vi "SWERVE_DRIVE_BEGIN.vi"(8 "error in":errorcluster) -> (0 "error out":errorcluster)   [LabVIEW 2023]
uses:
  <vilib>/Rock Robotics/WPI/ThirdParty/Phoenix-LabVIEW/Motor Controller/Controls/CTRE_Phoenix_MotorControl_TalonFXInvertType.ctl
  <vilib>/Rock Robotics/WPI/ThirdParty/Phoenix-LabVIEW/Pigeon IMU/CTRE_PigeonIMU_TareType.ctl
  <vilib>/Rock Robotics/WPI/ThirdParty/JAS_Junk/TrajLib/Trajectory_Library.lvlib
  SWERVE_DRIVE_GLOBALS.vi
  <vilib>/Rock Robotics/WPI/ThirdParty/JAS_Junk/TrajLib/Enum/DCMOTOR_TYPES_ENUM.ctl
  <vilib>/Rock Robotics/WPI/ThirdParty/Phoenix-LabVIEW/CANCoder/Controls/CTRE_Phoenix_CANcoder_StatusFrame.ctl
  <vilib>/Rock Robotics/WPI/ThirdParty/Phoenix-LabVIEW/CANCoder/Controls/CTRE_Phoenix_CANcoder_SensorInitializationStrategy.ctl
  <vilib>/Rock Robotics/WPI/ThirdParty/Phoenix-LabVIEW/Motor Controller/Controls/CTRE_Phoenix_MotorControl_FeedbackDevice_TalonFX.ctl
  <vilib>/Rock Robotics/WPI/ThirdParty/Phoenix-LabVIEW/Motor Controller/Controls/CTRE_Phoenix_MotorControl_NeutralMode.ctl
  <vilib>/Rock Robotics/WPI/ThirdParty/REV Robotics/REVLib/Typedef/Spark MAX Idle Mode.ctl
  <vilib>/Rock Robotics/WPI/ThirdParty/Phoenix-LabVIEW/Motor Controller/Controls/CTRE_Phoenix_MotorControl_StatorCurrentLimitConfiguration.ctl
  <vilib>/Analysis/Matrix/Datatypes/RealMatrix.ctl
  <vilib>/Analysis/Matrix/NI_Matrix.lvlib
  <vilib>/Rock Robotics/WPI/ThirdParty/Phoenix6/setters/TalonFX_SetSensorPosition.vi
  <vilib>/Rock Robotics/Network Tables/NT Write Variant.vi
  <vilib>/Rock Robotics/WPI/ThirdParty/JAS_Junk/TrajLib/TypeDef/DCMOTOR_SIM_SIMULATION_PARAMS.ctl
  <vilib>/Rock Robotics/WPI/ThirdParty/REV Robotics/REVLib/SubVI/Public/SPARK Open Brushless.vi
  <vilib>/Rock Robotics/WPI/ThirdParty/REV Robotics/REVLib/Typedef/Closed Loop Voltage Mode.ctl
  <vilib>/Rock Robotics/WPI/ThirdParty/REV Robotics/REVLib/Typedef/SPARK PID Gains.ctl
  <vilib>/Rock Robotics/WPI/ThirdParty/REV Robotics/REVLib/Typedef/SPARK Feedback Sensor.ctl
  <vilib>/Rock Robotics/WPI/ThirdParty/REV Robotics/REVLib/SubVI/Public/SPARK Configure Closed Loop MAXMotion.vi
  <vilib>/Rock Robotics/WPI/ThirdParty/REV Robotics/REVLib/SubVI/Public/SPARK Configure Closed Loop Voltage Mode.vi
  <vilib>/Rock Robotics/WPI/ThirdParty/REV Robotics/REVLib/SubVI/Public/SPARK Configure Closed Loop Gains.vi
  <vilib>/Rock Robotics/WPI/ThirdParty/REV Robotics/REVLib/SubVI/Public/SPARK Configure Basic Idle Mode.vi
  <vilib>/Rock Robotics/WPI/ThirdParty/REV Robotics/REVLib/SubVI/Public/SPARK Configure Closed Loop Basic.vi
  <vilib>/Rock Robotics/WPI/ThirdParty/REV Robotics/REVLib/SubVI/Public/SPARK Configure Power Smart Current Limit.vi
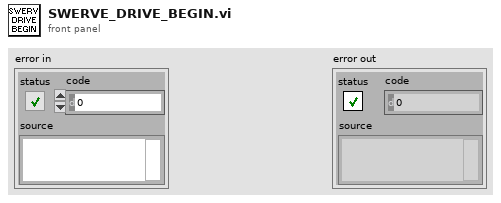
[diagram p1: front panel]
types:
  T1 = enum16{"Talon FX, P5", "Talon FX, P6", "SPARK MAX"}
  T2 = typedef "NI_Matrix.lvlib/RealMatrix.ctl" = dbl[][]
  T3 = typedef "CTRE_Phoenix_MotorControl_TalonFXInvertType.ctl" = enum16{"Counter-Clockwise", "Clockwise"}
  T4 = typedef "Trajectory_Library.lvlib/DCMOTOR_TYPES_ENUM.ctl" = enum16{"CIM", "AndyMark 9015", "Andy Mark RS 775 125", "Bag", "BaneBots RS 550", "BaneBots RS 775", "Falcon 500", "Mini CIM", "NEO", "NEO 550", "Romi BuiltIn", "Vex 775 Pro", "Snow Blower AM 2235A", "Bosch Seat AM 3493", "Falcon 500 FOC", "Kraken X60", "Kraken X60 FOC", "NEO Vortex"}
  T5 = typedef "Trajectory_Library.lvlib/DCMOTOR.CTL" = cluster{"nominalVoltage_Volts":dbl, "StallTorque_NM":dbl, "StallCurrent_Amps":dbl, "FreeCurrent_Amps":dbl, "FreeSpeed_RadPerSec":dbl, "R_Ohms":dbl, "KvINV_RadPerSecPerVolt":dbl, "Kt_NMPerAmp":dbl, "L_H":dbl, "Jr_KgM2":dbl}
  T6 = cluster{"Future Proof Configs":bool, "MotorOutputInverted":u16, "MotorOutputNeutralMode":u16, "MotorOutputDutyCycleNeutralDeadband":dbl, "MotorOutputPeakForwardDutyCycle":dbl, "MotorOutputPeakReverseDutyCycle":dbl, "MotorOutputControlTimesyncFreqHz":dbl, "CurrentLimitsStatorCurrentLimit":dbl, "CurrentLimitsStatorCurrentLimitEnable":bool, "CurrentLimitsSupplyCurrentLimit":dbl, "CurrentLimitsSupplyCurrentLimitEnable":bool, "CurrentLimitsSupplyCurrentLowerLimit":dbl, "CurrentLimitsSupplyCurrentLowerTime":dbl, "VoltageSupplyVoltageTimeConstant":dbl, "VoltagePeakForwardVoltage":dbl, "VoltagePeakReverseVoltage":dbl, "TorqueCurrentPeakForwardTorqueCurrent":dbl, "TorqueCurrentPeakReverseTorqueCurrent":dbl, "TorqueCurrentTorqueNeutralDeadband":dbl, "FeedbackFeedbackRotorOffset":dbl, "FeedbackSensorToMechanismRatio":dbl, "FeedbackRotorToSensorRatio":dbl, "FeedbackFeedbackSensorSource":u16, "FeedbackFeedbackRemoteSensorID":i16, "FeedbackVelocityFilterTimeConstant":dbl, "DifferentialSensorsDifferentialSensorSource":u16, "DifferentialSensorsDifferentialTalonFXSensorID":i16, "DifferentialSensorsDifferentialRemoteSensorID":i16, "DifferentialConstantsPeakDifferentialDutyCycle":dbl, "DifferentialConstantsPeakDifferentialVoltage":dbl, "DifferentialConstantsPeakDifferentialTorqueCurrent":dbl, "OpenLoopRampsDutyCycleOpenLoopRampPeriod":dbl, "OpenLoopRampsVoltageOpenLoopRampPeriod":dbl, "OpenLoopRampsTorqueOpenLoopRampPeriod":dbl, "ClosedLoopRampsDutyCycleClosedLoopRampPeriod":dbl, "ClosedLoopRampsVoltageClosedLoopRampPeriod":dbl, "ClosedLoopRampsTorqueClosedLoopRampPeriod":dbl, "HardwareLimitSwitchForwardLimitType":u16, "HardwareLimitSwitchForwardLimitAutosetPositionEnable":bool, "HardwareLimitSwitchForwardLimitAutosetPositionValue":dbl, "HardwareLimitSwitchForwardLimitEnable":bool, "HardwareLimitSwitchForwardLimitSource":u16, "HardwareLimitSwitchForwardLimitRemoteSensorID":i16, "HardwareLimitSwitchReverseLimitType":u16, "HardwareLimitSwitchReverseLimitAutosetPositionEnable":bool, "HardwareLimitSwitchReverseLimitAutosetPositionValue":dbl, "HardwareLimitSwitchReverseLimitEnable":bool, "HardwareLimitSwitchReverseLimitSource":u16, "HardwareLimitSwitchReverseLimitRemoteSensorID":i16, "AudioBeepOnBoot":bool, "AudioBeepOnConfig":bool, "AudioAllowMusicDurDisable":bool, "SoftwareLimitSwitchForwardSoftLimitEnable":bool, "SoftwareLimitSwitchReverseSoftLimitEnable":bool, "SoftwareLimitSwitchForwardSoftLimitThreshold":dbl, "SoftwareLimitSwitchReverseSoftLimitThreshold":dbl, "MotionMagicMotionMagicCruiseVelocity":dbl, "MotionMagicMotionMagicAcceleration":dbl, "MotionMagicMotionMagicJerk":dbl, "MotionMagicMotionMagicExpo_kV":dbl, "MotionMagicMotionMagicExpo_kA":dbl, "CustomParamsCustomParam0":i16, "CustomParamsCustomParam1":i16, "ClosedLoopGeneralContinuousWrap":bool, "Slot0kP":dbl, "Slot0kI":dbl, "Slot0kD":dbl, "Slot0kS":dbl, "Slot0kV":dbl, "Slot0kA":dbl, "Slot0kG":dbl, "Slot0GravityType":u16, "Slot0StaticFeedforwardSign":u16, "Slot1kP":dbl, "Slot1kI":dbl, "Slot1kD":dbl, "Slot1kS":dbl, "Slot1kV":dbl, "Slot1kA":dbl, "Slot1kG":dbl, "Slot1GravityType":u16, "Slot1StaticFeedforwardSign":u16, "Slot2kP":dbl, "Slot2kI":dbl, "Slot2kD":dbl, "Slot2kS":dbl, "Slot2kV":dbl, "Slot2kA":dbl, "Slot2kG":dbl, "Slot2GravityType":u16, "Slot2StaticFeedforwardSign":u16}
  T7 = typedef "Trajectory_Library.lvlib/DCMOTOR_SIM_SIMULATION_PARAMS.ctl" = cluster{"Pos Sim Std Dev Rotations":dbl, "Vel Sim Std Dev RPM":dbl}
  T8 = typedef "CTRE_Phoenix_MotorControl_StatorCurrentLimitConfiguration.ctl" = cluster{"Enable?":bool, "Current Limit":dbl, "Threshold Current":dbl, "Threshold Time":dbl}
  T9 = typedef "CTRE_Phoenix_MotorControl_NeutralMode.ctl" = enum8{"EEPROMSetting", "Override to Coast", "Override to Brake"}
  T10 = typedef "SPARK Feedback Sensor.ctl" = enum16{"No Sensor", "Primary Encoder", "Analog Sensor", "Alternate or External Encoder", "Duty Cycle Sensor"}
  T11 = typedef "Spark MAX Idle Mode.ctl" = enum16{"Coast", "Brake"}
  T12 = typedef "SPARK PID Gains.ctl" = cluster{"kP":dbl, "kI":dbl, "kD":dbl}
  T13 = typedef "Closed Loop Voltage Mode.ctl" = enum16{"Disabled", "Voltage Output", "Voltage Compensation"}
  T14 = typedef "CTRE_Phoenix_CANcoder_SensorInitializationStrategy.ctl" = enum16{"Boot To Zero", "Boot To Absolute Position"}
  T15 = typedef "Trajectory_Library.lvlib/LINEAR_SYSTEM.ctl" = cluster{"m_A":T2, "m_B":T2, "m_C":T2, "m_D":T2, "States":i32, "Inputs":i32, "Outputs":i32}
  T16 = typedef "Trajectory_Library.lvlib/DCMOTOR_SIM.ctl" = cluster{"LinearSystemSim":T17, "GearBox":T5, "Gearing":dbl}
  T17 = typedef "Trajectory_Library.lvlib/LINEAR_SYSTEM_SIM.ctl" = cluster{"m_Plant":T15, "m_X":T2, "m_Y":T2, "m_U":T2, "MeasureStdDev":T2}
  T18 = typedef "CTRE_PigeonIMU_TareType.ctl" = u8
  T19 = typedef "CTRE_Phoenix_MotorControl_FeedbackDevice_TalonFX.ctl" = i8
  T20 = typedef "WPI_MotorControlDeviceRef.ctl" = cluster{"DeviceStatus":errorcluster, "Type":T21, "PWM":cluster{"PWM Channel":T22, "DeadBand":T23}, "CAN":cluster{"Device Number":u8, "SetOutput VI Ref":variant, "GetOutput VI Ref":variant, "Enable VI Ref":variant, "Disable VI Ref":variant, "Data":variant}, "Invert":bool, "DIO PWM":cluster{"PWM \"Enable\" Channel":T22, "DIOChannel":T24, "PWM Rate":dbl}}
  T21 = typedef "WPI_MotorControlType.ctl" = enum16{"PWM", "CAN", "DIO PWM"}
  T22 = typedef "FPGA_DIOPWMChannel.ctl" = enum8{"PWM 0", "PWM 1", "PWM 2", "PWM 3", "PWM 4", "PWM 5", "PWM 6", "PWM 7", "PWM 8", "PWM 9", "PWM MXP 0", "PWM MXP 1", "PWM MXP 2", "PWM MXP 3", "PWM MXP 4", "PWM MXP 5", "PWM MXP 6", "PWM MXP 7", "PWM MXP 8", "PWM MXP 9", "Invalid"}
  T23 = typedef "WPI_PWMDeadband.ctl" = cluster{"Name":string, "maxPositivePwm":i32, "minPositivePwm":i32, "centerPwm":i32, "maxNegativePwm":i32, "minNegativePwm":i32, "angularRange":u16}
  T24 = typedef "FPGA_DIOChannel.ctl" = enum8{"DIO 0", "DIO 1", "DIO 2", "DIO 3", "DIO 4", "DIO 5", "DIO 6", "DIO 7", "DIO 8", "DIO 9", "DIO MXP 0", "DIO MXP 1", "DIO MXP 2", "DIO MXP 3", "DIO MXP 4", "DIO MXP 5", "DIO MXP 6", "DIO MXP 7", "DIO MXP 8", "DIO MXP 9", "DIO MXP 10", "DIO MXP 11", "DIO MXP 12", "DIO MXP 13", "DIO MXP 14", "DIO MXP 15", "SPI Port CS1", "SPI Port CS2", "SPI Port CS3", "SPI Port MISO", "SPI Port MOSI", "Invalid"}
  T25 = typedef "DeviceReference.ctl" = cluster{"CANbus Name":string, "Device Encoding":u32, "Device Name":string}
  T26 = typedef "CTRE_Phoenix_CANcoder_StatusFrame.ctl" = u32
  T27 = typedef "CTRE_Phoenix_CANcoder_DeviceRef.ctl" = cluster{"DeviceStatus":errorcluster, "Device Number":u8, "Handle":u64, "UsageFrame":u32, "Library Path":path}
  T28 = typedef "CTRE_PigeonIMU_DeviceRef.ctl" = cluster{"DeviceStatus":errorcluster, "Device Number":u8, "Type":T29, "Device ID":u32, "Handle":u64, "UsageFrame":u32, "Library Path":path}
  T29 = typedef "CTRE_PigeonIMU_ConnectionType.ctl" = u32
  T30 = typedef "Trajectory_Library.lvlib/TRANSLATION2D.ctl" = cluster{"X":dbl, "Y":dbl}
  T31 = typedef "Trajectory_Library.lvlib/SWERVE_DRIVE_KINEMATICS.ctl" = cluster{"NumModules":i32, "InverseKinematics":T2, "ForwardKinematics":T2, "Modules":T30[], "PrevCoR":T30, "SavedModuleStates":T32[]}
  T32 = typedef "Trajectory_Library.lvlib/SWERVE_DRIVE_MODULE_STATE.ctl" = cluster{"Speed":dbl, "Angle":T33}
  T33 = typedef "Trajectory_Library.lvlib/ROTATION2D.ctl" = cluster{"VALUE":dbl, "COS":dbl, "SIN":dbl}
  T34 = typedef "Trajectory_Library.lvlib/SWERVE_DRIVE_MODULE_POSITION.ctl" = cluster{"Distance":dbl, "Angle":T33, "P":bool}
  T35 = typedef "Trajectory_Library.lvlib/POSE2D.ctl" = cluster{"TRANSLATION":T30, "ROTATION":T33}
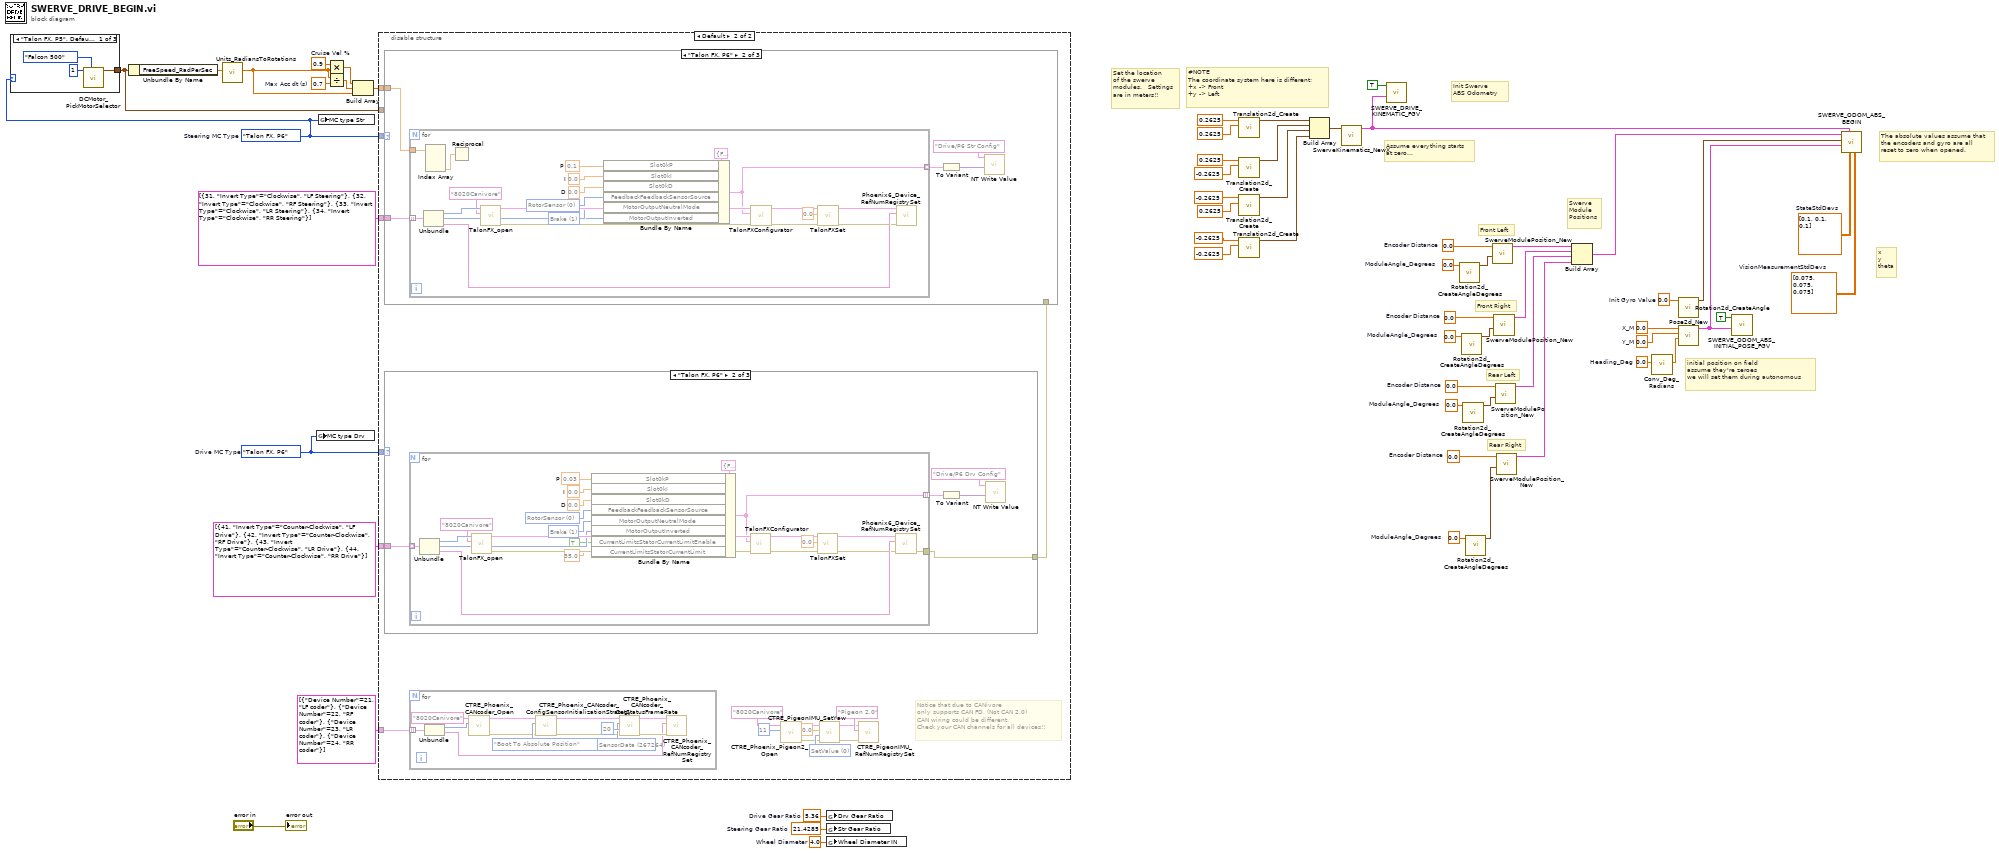
[diagram p0: block diagram]
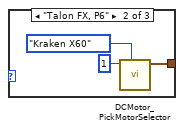
[diagram p2: hidden frame]
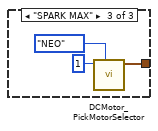
[diagram p3: hidden frame]
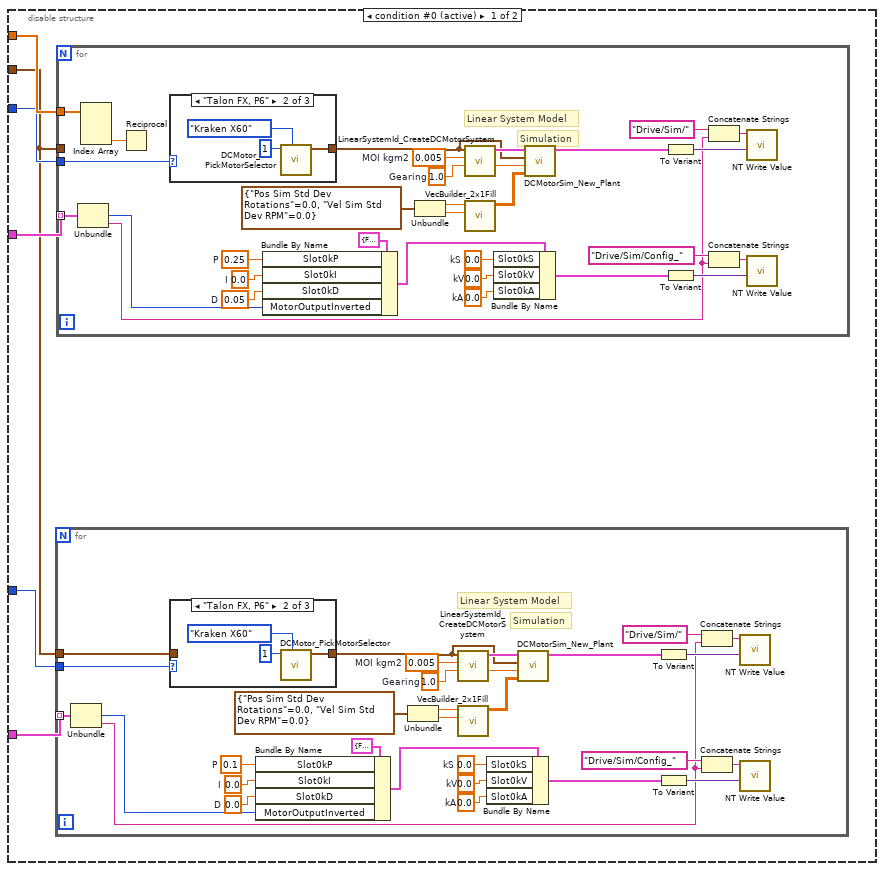
[diagram p4: hidden frame]
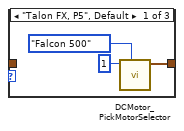
[diagram p5: hidden frame]
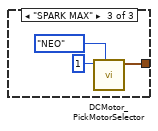
[diagram p6: hidden frame]
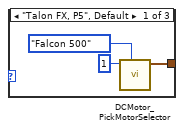
[diagram p7: hidden frame]
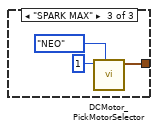
[diagram p8: hidden frame]
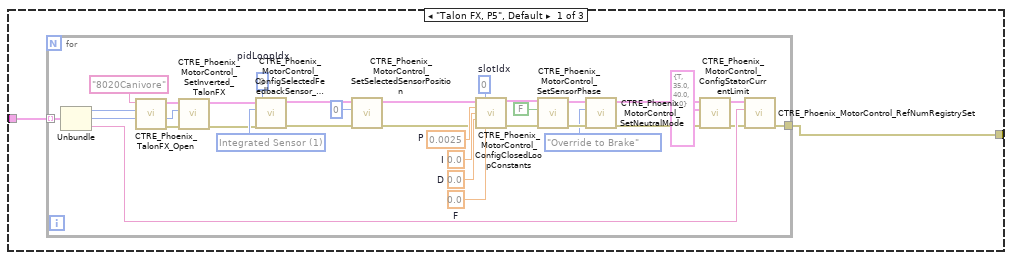
[diagram p9: hidden frame]
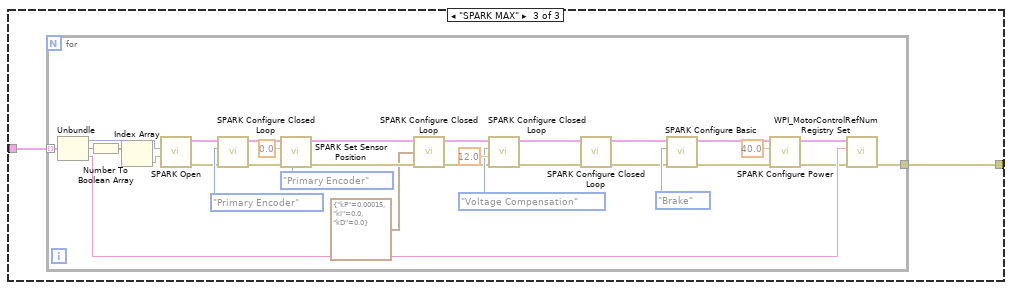
[diagram p10: hidden frame]
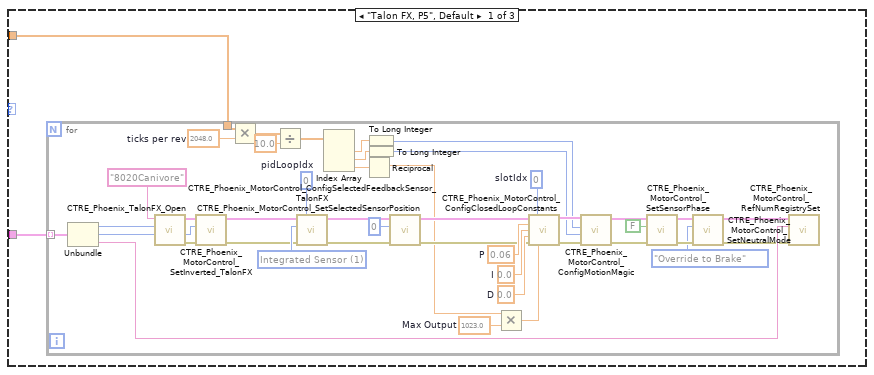
[diagram p11: hidden frame]
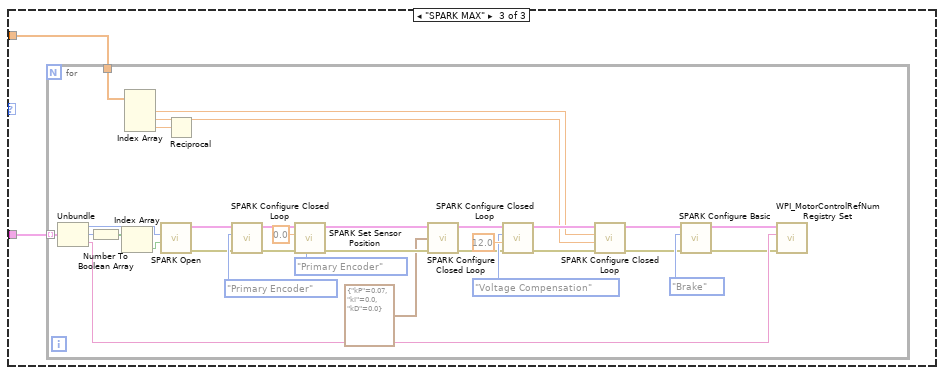
[diagram p12: hidden frame]
diagram:
  w3 = 4.0  # Wheel Diameter
  w5 = T1."Talon FX, P6"  # Drive MC Type
  w1 = T1."Talon FX, P6"  # Steering MC Type
  w9 = 0.7  # Max Acc dt (s)
  w8 = 0.9  # Cruise Vel %
  w55 = T2 [[0.075], [0.075], [0.075]]  # VisionMeasurementStdDevs
  w54 = T2 [[0.1], [0.1], [0.1]]  # StateStdDevs
  w50 = 0.0  # Init Gyro Value
  w51 = 0.0  # Heading_Deg
  w49 = 0.0  # Y_M
  w48 = 0.0  # X_M
  w35 = 0.0  # ModuleAngle_Degrees
  w37 = 0.0  # Encoder Distance
  w38 = 0.0  # ModuleAngle_Degrees
  w40 = 0.0  # Encoder Distance
  w41 = 0.0  # ModuleAngle_Degrees
  w43 = 0.0  # Encoder Distance
  w45 = 0.0  # ModuleAngle_Degrees
  w47 = 0.0  # Encoder Distance
  w4 = 21.4285  # Steering Gear Ratio
  w28 = 5.36  # Drive Gear Ratio
  # "x\ny\ntheta"
  # "Init Swerve\nABS Odometry"
  # "initial position on field\nassume they're zeroes\nwe will set them during autonomous"
  # "The absolute values assume that\nthe encoders and gyro are all\nreset to zero when opened."
  # "Assume everything starts\nat zero..."
  # "Front Left"
  # "Swerve\nModule\nPositions"
  # "Rear Right"
  # "Rear Left"
  # "Front Right"
  # "#NOTE\nThe coordinate system here is different;\n+x -> Front\n+y -> Left"
  # "Set the location\nof the swerve \nmodules.   Settings\nare in meters!!"
  n1 = case shown="\"Talon FX, P5\", Default" w1 {
    tunnel: [w61 w64 w67] -> w2
    frame "Talon FX, P5", Default {
      n2 = call <vilib>:"DCMotor_PickMotorSelector.vi"("DCMOTOR_TYPES"=DCMOTOR_TYPES_ENUM."Falcon 500", "Num Motors"=1) -> ("DCMOTOR"=w61:T5)  [unwired: 9 in]
    }
    frame "Talon FX, P6" {
      n3 = call <vilib>:"DCMotor_PickMotorSelector.vi"("DCMOTOR_TYPES"=DCMOTOR_TYPES_ENUM."Kraken X60", "Num Motors"=1) -> ("DCMOTOR"=w64:T5)  [unwired: 9 in]
    }
    frame "SPARK MAX" {
      n4 = call <vilib>:"DCMotor_PickMotorSelector.vi"("DCMOTOR_TYPES"=DCMOTOR_TYPES_ENUM."NEO", "Num Motors"=1) -> ("DCMOTOR"=w67:T5)  [unwired: 9 in]
    }
  }
  n5 = Unbundle By Name(w2) -> ("FreeSpeed_RadPerSec"=w29:dbl)
  n6 = call <vilib>:"Units_RadiansToRotations.vi"("Radians"=w29) -> ("Rotations"=w7:dbl)  [unwired: 10 in]
  n7 = global write "SWERVE_DRIVE_GLOBALS.vi" "MC type Drv"(w5) -> ()
  n8 = global write "SWERVE_DRIVE_GLOBALS.vi" "MC type Str"(w1) -> ()
  n9 = Multiply(x=w8, y=w7) -> (x*y=w10:dbl)
  n10 = Divide(x=w7, y=w9) -> (x/y=w11:dbl)
  n11 = Build Array(w10, w11, w7) -> (w6:dbl[])
  n12 = disable-structure shown="Default" {
    disable-tunnel: cluster{i32, "Invert Type":T3, string}[] [{31, "Invert Type"=enum."Clockwise", "LF Steering"}, {32, "Invert Type"=enum."Clockwise", "RF Steering"}, {33, "Invert Type"=enum."Clockwise", "LR Steering"}, {34, "Invert Type"=enum."Clockwise", "RR Steering"}] ("Array") -> [w74 w166]
    disable-tunnel: cluster{"Device Number":u8, string}[] [{"Device Number"=21, "LF coder"}, {"Device Number"=22, "RF coder"}, {"Device Number"=23, "LR coder"}, {"Device Number"=24, "RR coder"}] ("CANcoder ref") -> [_ w165]
    disable-tunnel: cluster{i32, "Invert Type":T3, string}[] [{41, "Invert Type"=enum."Counter-Clockwise", "LF Drive"}, {42, "Invert Type"=enum."Counter-Clockwise", "RF Drive"}, {43, "Invert Type"=enum."Counter-Clockwise", "LR Drive"}, {44, "Invert Type"=enum."Counter-Clockwise", "RR Drive"}] ("Array") -> [w73 w155]
    disable-tunnel: w6 -> [w72 w154]
    disable-tunnel: w5 -> [w70 w153]
    disable-tunnel: w1 -> [w71 w152]
    disable-tunnel: w2 -> [w69 _]
    frame condition #0 (active) {
      n13 = for {
        tunnel: w73 -> [w78] mode=indexing
        tunnel: w70 -> [w77]
        tunnel: w69 -> [w76]
        w84 = 0.0  # kA
        w85 = 0.0  # kV
        w86 = 0.0  # kS
        w89 = 0.0  # D
        w90 = 0.0  # I
        w91 = 0.1  # P
        w95 = 1.0  # Gearing
        w94 = 0.005  # MOI kgm2
        # "Simulation"
        # "Linear System Model"
        n14 = Unbundle(w78) -> ("Invert Type"=w88:T3, w79:string)  [unwired: 1 out]
        n15 = case shown="\"Talon FX, P6\"" w77 {
          tunnel: w76 -> [_ _ _]
          tunnel: [w105 w108 w111] -> w93
          frame "Talon FX, P5", Default {
            n16 = call <vilib>:"DCMotor_PickMotorSelector.vi"("DCMOTOR_TYPES"=DCMOTOR_TYPES_ENUM."Falcon 500", "Num Motors"=1) -> ("DCMOTOR"=w105:T5)  [unwired: 9 in]
          }
          frame "Talon FX, P6" {
            n17 = call <vilib>:"DCMotor_PickMotorSelector.vi"("DCMOTOR_TYPES"=DCMOTOR_TYPES_ENUM."Kraken X60", "Num Motors"=1) -> ("DCMOTOR"=w108:T5)  [unwired: 9 in]
          }
          frame "SPARK MAX" {
            n18 = call <vilib>:"DCMotor_PickMotorSelector.vi"("DCMOTOR_TYPES"=DCMOTOR_TYPES_ENUM."NEO", "Num Motors"=1) -> ("DCMOTOR"=w111:T5)  [unwired: 9 in]
          }
        }
        n19 = Bundle By Name(cluster=T6 {"Future Proof Configs"=FALSE, "MotorOutputInverted"=0, "MotorOutputNeutralMode"=0, "MotorOutputDutyCycleNeutralDeadband"=0.0, "MotorOutputPeakForwardDutyCycle"=1.0, "MotorOutputPeakReverseDutyCycle"=-1.0, "MotorOutputControlTimesyncFreqHz"=0.0, "CurrentLimitsStatorCurrentLimit"=120.0, "CurrentLimitsStatorCurrentLimitEnable"=TRUE, "CurrentLimitsSupplyCurrentLimit"=70.0, "CurrentLimitsSupplyCurrentLimitEnable"=TRUE, "CurrentLimitsSupplyCurrentLowerLimit"=40.0, "CurrentLimitsSupplyCurrentLowerTime"=1.0, "VoltageSupplyVoltageTimeConstant"=0.0, "VoltagePeakForwardVoltage"=16.0, "VoltagePeakReverseVoltage"=-16.0, "TorqueCurrentPeakForwardTorqueCurrent"=800.0, "TorqueCurrentPeakReverseTorqueCurrent"=-800.0, "TorqueCurrentTorqueNeutralDeadband"=0.0, "FeedbackFeedbackRotorOffset"=0.0, "FeedbackSensorToMechanismRatio"=1.0, "FeedbackRotorToSensorRatio"=1.0, "FeedbackFeedbackSensorSource"=0, "FeedbackFeedbackRemoteSensorID"=0, "FeedbackVelocityFilterTimeConstant"=0.0, "DifferentialSensorsDifferentialSensorSource"=0, "DifferentialSensorsDifferentialTalonFXSensorID"=0, "DifferentialSensorsDifferentialRemoteSensorID"=0, "DifferentialConstantsPeakDifferentialDutyCycle"=2.0, "DifferentialConstantsPeakDifferentialVoltage"=32.0, "DifferentialConstantsPeakDifferentialTorqueCurrent"=1600.0, "OpenLoopRampsDutyCycleOpenLoopRampPeriod"=0.0, "OpenLoopRampsVoltageOpenLoopRampPeriod"=0.0, "OpenLoopRampsTorqueOpenLoopRampPeriod"=0.0, "ClosedLoopRampsDutyCycleClosedLoopRampPeriod"=0.0, "ClosedLoopRampsVoltageClosedLoopRampPeriod"=0.0, "ClosedLoopRampsTorqueClosedLoopRampPeriod"=0.0, "HardwareLimitSwitchForwardLimitType"=0, "HardwareLimitSwitchForwardLimitAutosetPositionEnable"=FALSE, "HardwareLimitSwitchForwardLimitAutosetPositionValue"=0.0, "HardwareLimitSwitchForwardLimitEnable"=TRUE, "HardwareLimitSwitchForwardLimitSource"=0, "HardwareLimitSwitchForwardLimitRemoteSensorID"=0, "HardwareLimitSwitchReverseLimitType"=0, "HardwareLimitSwitchReverseLimitAutosetPositionEnable"=FALSE, "HardwareLimitSwitchReverseLimitAutosetPositionValue"=0.0, "HardwareLimitSwitchReverseLimitEnable"=TRUE, "HardwareLimitSwitchReverseLimitSource"=0, "HardwareLimitSwitchReverseLimitRemoteSensorID"=0, "AudioBeepOnBoot"=TRUE, "AudioBeepOnConfig"=TRUE, "AudioAllowMusicDurDisable"=FALSE, "SoftwareLimitSwitchForwardSoftLimitEnable"=FALSE, "SoftwareLimitSwitchReverseSoftLimitEnable"=FALSE, "SoftwareLimitSwitchForwardSoftLimitThreshold"=0.0, "SoftwareLimitSwitchReverseSoftLimitThreshold"=0.0, "MotionMagicMotionMagicCruiseVelocity"=0.0, "MotionMagicMotionMagicAcceleration"=0.0, "MotionMagicMotionMagicJerk"=0.0, "MotionMagicMotionMagicExpo_kV"=0.12, "MotionMagicMotionMagicExpo_kA"=0.1, "CustomParamsCustomParam0"=0, "CustomParamsCustomParam1"=0, "ClosedLoopGeneralContinuousWrap"=FALSE, "Slot0kP"=0.0, "Slot0kI"=0.0, "Slot0kD"=0.0, "Slot0kS"=0.0, "Slot0kV"=0.0, "Slot0kA"=0.0, "Slot0kG"=0.0, "Slot0GravityType"=0, "Slot0StaticFeedforwardSign"=0, "Slot1kP"=0.0, "Slot1kI"=0.0, "Slot1kD"=0.0, "Slot1kS"=0.0, "Slot1kV"=0.0, "Slot1kA"=0.0, "Slot1kG"=0.0, "Slot1GravityType"=0, "Slot1StaticFeedforwardSign"=0, "Slot2kP"=0.0, "Slot2kI"=0.0, "Slot2kD"=0.0, "Slot2kS"=0.0, "Slot2kV"=0.0, "Slot2kA"=0.0, "Slot2kG"=0.0, "Slot2GravityType"=0, "Slot2StaticFeedforwardSign"=0} ("DeviceConfiguration"), "Slot0kP"=w91, "Slot0kI"=w90, "Slot0kD"=w89, "MotorOutputInverted"=w88) -> (w87:T6)
        n20 = Unbundle(T7 {"Pos Sim Std Dev Rotations"=0.0, "Vel Sim Std Dev RPM"=0.0} ("DCMOTORSim_Simulation_Params")) -> ("Pos Sim Std Dev Rotations"=w100:dbl, "Vel Sim Std Dev RPM"=w99:dbl)
        n21 = call <vilib>:"LinearSystemId_CreateDCMotorSystem.vi"("G"=w95, "jKgMetersSquared"=w94, "DCMOTOR"=w93) -> ("Linearsystem"=w103:T15)  [unwired: 7 in, 1 out]
        n22 = call <vilib>:"VecBuilder_2x1Fill.vi"("R1"=w99, "R0"=w100) -> ("output matrix"=w102:T2)  [unwired: 9 in]
        n23 = Bundle By Name(cluster=w87, "Slot0kS"=w86, "Slot0kV"=w85, "Slot0kA"=w84) -> (w80:T6)
        n24 = call <vilib>:"DCMotorSim_New_Plant.vi"("MeasurementStdDev"=w102, "Gearing"=w95, "GearBox"=w93, "Plant"=w103) -> ("DCMotorSim"=w92:T16)  [unwired: 6 in, 1 out]
        n25 = To Variant(anything=w92) -> (Variant=w98:variant)
        n26 = To Variant(anything=w80) -> (Variant=w81:variant)
        n27 = Concatenate Strings("Drive/Sim/" ("name"), w79) -> (w97:string)
        n28 = Concatenate Strings("Drive/Sim/Config_" ("name"), w79) -> (w82:string)
        n29 = call-poly <vilib>:"NT Write Value.vi"("variant"=w98, "name"=w97) -> ()  [unwired: 9 in, 1 out]
        n30 = call-poly <vilib>:"NT Write Value.vi"("variant"=w81, "name"=w82) -> ()  [unwired: 9 in, 1 out]
      }
      n31 = for {
        tunnel: w74 -> [w142] mode=indexing
        tunnel: w72 -> [w140]
        tunnel: w69 -> [_]
        tunnel: w71 -> [w113]
        w121 = 0.0  # kA
        w122 = 0.0  # kV
        w123 = 0.0  # kS
        w126 = 0.05  # D
        w127 = 0.0  # I
        w128 = 0.25  # P
        w131 = 1.0  # Gearing
        w130 = 0.005  # MOI kgm2
        # "Simulation"
        # "Linear System Model"
        n32 = Unbundle(w142) -> ("Invert Type"=w125:T3, w116:string)  [unwired: 1 out]
        n33 = Index Array(array=w140) -> (element #3=w141:dbl)  [unwired: 3 in, 2 out]
        n34 = Reciprocal(x=w141) -> ()  [unwired: 1 out]
        n35 = case shown="\"Talon FX, P6\"" w113 {
          tunnel: [w144 w147 w150] -> w114
          frame "Talon FX, P5", Default {
            n36 = call <vilib>:"DCMotor_PickMotorSelector.vi"("DCMOTOR_TYPES"=DCMOTOR_TYPES_ENUM."Falcon 500", "Num Motors"=1) -> ("DCMOTOR"=w144:T5)  [unwired: 9 in]
          }
          frame "Talon FX, P6" {
            n37 = call <vilib>:"DCMotor_PickMotorSelector.vi"("DCMOTOR_TYPES"=DCMOTOR_TYPES_ENUM."Kraken X60", "Num Motors"=1) -> ("DCMOTOR"=w147:T5)  [unwired: 9 in]
          }
          frame "SPARK MAX" {
            n38 = call <vilib>:"DCMotor_PickMotorSelector.vi"("DCMOTOR_TYPES"=DCMOTOR_TYPES_ENUM."NEO", "Num Motors"=1) -> ("DCMOTOR"=w150:T5)  [unwired: 9 in]
          }
        }
        n39 = Bundle By Name(cluster=T6 {"Future Proof Configs"=FALSE, "MotorOutputInverted"=0, "MotorOutputNeutralMode"=0, "MotorOutputDutyCycleNeutralDeadband"=0.0, "MotorOutputPeakForwardDutyCycle"=1.0, "MotorOutputPeakReverseDutyCycle"=-1.0, "MotorOutputControlTimesyncFreqHz"=0.0, "CurrentLimitsStatorCurrentLimit"=120.0, "CurrentLimitsStatorCurrentLimitEnable"=TRUE, "CurrentLimitsSupplyCurrentLimit"=70.0, "CurrentLimitsSupplyCurrentLimitEnable"=TRUE, "CurrentLimitsSupplyCurrentLowerLimit"=40.0, "CurrentLimitsSupplyCurrentLowerTime"=1.0, "VoltageSupplyVoltageTimeConstant"=0.0, "VoltagePeakForwardVoltage"=16.0, "VoltagePeakReverseVoltage"=-16.0, "TorqueCurrentPeakForwardTorqueCurrent"=800.0, "TorqueCurrentPeakReverseTorqueCurrent"=-800.0, "TorqueCurrentTorqueNeutralDeadband"=0.0, "FeedbackFeedbackRotorOffset"=0.0, "FeedbackSensorToMechanismRatio"=1.0, "FeedbackRotorToSensorRatio"=1.0, "FeedbackFeedbackSensorSource"=0, "FeedbackFeedbackRemoteSensorID"=0, "FeedbackVelocityFilterTimeConstant"=0.0, "DifferentialSensorsDifferentialSensorSource"=0, "DifferentialSensorsDifferentialTalonFXSensorID"=0, "DifferentialSensorsDifferentialRemoteSensorID"=0, "DifferentialConstantsPeakDifferentialDutyCycle"=2.0, "DifferentialConstantsPeakDifferentialVoltage"=32.0, "DifferentialConstantsPeakDifferentialTorqueCurrent"=1600.0, "OpenLoopRampsDutyCycleOpenLoopRampPeriod"=0.0, "OpenLoopRampsVoltageOpenLoopRampPeriod"=0.0, "OpenLoopRampsTorqueOpenLoopRampPeriod"=0.0, "ClosedLoopRampsDutyCycleClosedLoopRampPeriod"=0.0, "ClosedLoopRampsVoltageClosedLoopRampPeriod"=0.0, "ClosedLoopRampsTorqueClosedLoopRampPeriod"=0.0, "HardwareLimitSwitchForwardLimitType"=0, "HardwareLimitSwitchForwardLimitAutosetPositionEnable"=FALSE, "HardwareLimitSwitchForwardLimitAutosetPositionValue"=0.0, "HardwareLimitSwitchForwardLimitEnable"=TRUE, "HardwareLimitSwitchForwardLimitSource"=0, "HardwareLimitSwitchForwardLimitRemoteSensorID"=0, "HardwareLimitSwitchReverseLimitType"=0, "HardwareLimitSwitchReverseLimitAutosetPositionEnable"=FALSE, "HardwareLimitSwitchReverseLimitAutosetPositionValue"=0.0, "HardwareLimitSwitchReverseLimitEnable"=TRUE, "HardwareLimitSwitchReverseLimitSource"=0, "HardwareLimitSwitchReverseLimitRemoteSensorID"=0, "AudioBeepOnBoot"=TRUE, "AudioBeepOnConfig"=TRUE, "AudioAllowMusicDurDisable"=FALSE, "SoftwareLimitSwitchForwardSoftLimitEnable"=FALSE, "SoftwareLimitSwitchReverseSoftLimitEnable"=FALSE, "SoftwareLimitSwitchForwardSoftLimitThreshold"=0.0, "SoftwareLimitSwitchReverseSoftLimitThreshold"=0.0, "MotionMagicMotionMagicCruiseVelocity"=0.0, "MotionMagicMotionMagicAcceleration"=0.0, "MotionMagicMotionMagicJerk"=0.0, "MotionMagicMotionMagicExpo_kV"=0.12, "MotionMagicMotionMagicExpo_kA"=0.1, "CustomParamsCustomParam0"=0, "CustomParamsCustomParam1"=0, "ClosedLoopGeneralContinuousWrap"=FALSE, "Slot0kP"=0.0, "Slot0kI"=0.0, "Slot0kD"=0.0, "Slot0kS"=0.0, "Slot0kV"=0.0, "Slot0kA"=0.0, "Slot0kG"=0.0, "Slot0GravityType"=0, "Slot0StaticFeedforwardSign"=0, "Slot1kP"=0.0, "Slot1kI"=0.0, "Slot1kD"=0.0, "Slot1kS"=0.0, "Slot1kV"=0.0, "Slot1kA"=0.0, "Slot1kG"=0.0, "Slot1GravityType"=0, "Slot1StaticFeedforwardSign"=0, "Slot2kP"=0.0, "Slot2kI"=0.0, "Slot2kD"=0.0, "Slot2kS"=0.0, "Slot2kV"=0.0, "Slot2kA"=0.0, "Slot2kG"=0.0, "Slot2GravityType"=0, "Slot2StaticFeedforwardSign"=0} ("DeviceConfiguration"), "Slot0kP"=w128, "Slot0kI"=w127, "Slot0kD"=w126, "MotorOutputInverted"=w125) -> (w124:T6)
        n40 = Unbundle(T7 {"Pos Sim Std Dev Rotations"=0.0, "Vel Sim Std Dev RPM"=0.0} ("DCMOTORSim_Simulation_Params")) -> ("Pos Sim Std Dev Rotations"=w136:dbl, "Vel Sim Std Dev RPM"=w135:dbl)
        n41 = call <vilib>:"LinearSystemId_CreateDCMotorSystem.vi"("G"=w131, "jKgMetersSquared"=w130, "DCMOTOR"=w114) -> ("Linearsystem"=w139:T15)  [unwired: 7 in, 1 out]
        n42 = call <vilib>:"VecBuilder_2x1Fill.vi"("R1"=w135, "R0"=w136) -> ("output matrix"=w138:T2)  [unwired: 9 in]
        n43 = Bundle By Name(cluster=w124, "Slot0kS"=w123, "Slot0kV"=w122, "Slot0kA"=w121) -> (w117:T6)
        n44 = call <vilib>:"DCMotorSim_New_Plant.vi"("MeasurementStdDev"=w138, "Gearing"=w131, "GearBox"=w114, "Plant"=w139) -> ("DCMotorSim"=w129:T16)  [unwired: 6 in, 1 out]
        n45 = To Variant(anything=w129) -> (Variant=w134:variant)
        n46 = To Variant(anything=w117) -> (Variant=w118:variant)
        n47 = Concatenate Strings("Drive/Sim/" ("name"), w116) -> (w133:string)
        n48 = Concatenate Strings("Drive/Sim/Config_" ("name"), w116) -> (w119:string)
        n49 = call-poly <vilib>:"NT Write Value.vi"("variant"=w134, "name"=w133) -> ()  [unwired: 9 in, 1 out]
        n50 = call-poly <vilib>:"NT Write Value.vi"("variant"=w118, "name"=w119) -> ()  [unwired: 9 in, 1 out]
      }
    }
    frame condition #1 {
      w159 = T18 0 items=["SetValue"=0, "AddOffset"=1, "MatchCompass"=2, "SetOffset"=255] ("TareType (SetValue)")
      # "Notice that due to CANivore \nonly supports CAN FD, (Not CAN 2.0) \nCAN wiring could be different.\nCheck your CAN channels for all devices!!"
      n51 = case shown="\"Talon FX, P6\"" w153 {
        tunnel: w155 -> [w169 w207 w229]
        tunnel: [w168 w206 w228] -> w167
        frame "Talon FX, P5", Default {
          n52 = for {
            tunnel: w169 -> [w202] mode=indexing
            tunnel: [w170] -> w168
            w192 = 0  # slotIdx
            w193 = 0.0  # F
            w185 = 0.0  # D
            w186 = 0.0  # I
            w187 = 0.0025  # P
            w200 = 0  # pidLoopIdx
            w201 = T19 1 items=["Integrated Sensor"=1, "Sensor Sum (S0 + S1)"=9, "Sensor Difference (D0 - D1)"=10, "Remote Source 0"=11, "Remote Source 1"=12, "None"=14, "Software Emulated"=15] ("Talon FX Feedback Device")
            n53 = Unbundle(w202) -> (w198:i32, "Invert Type"=w178:T3, w199:string)
            n54 = call <vilib>:"CTRE_Phoenix_TalonFX_Open.vi"("Device Number"=w198, "CAN Bus"="8020Canivore") -> ("error out"=w181:errorcluster, "PhoenixMotorControlDevRef"=w184:T20)  [unwired: 8 in]
            n55 = call <vilib>:"CTRE_Phoenix_MotorControl_SetInverted_TalonFX.vi"("error in (no error)"=w181, "Invert Type"=w178, "PhoenixMotorControlDevRef"=w184) -> ("error out"=w182:errorcluster, "PhoenixMotorControlDevRef"=w183:T20)  [unwired: 7 in]
            n56 = call <vilib>:"CTRE_Phoenix_MotorControl_ConfigSelectedFeedbackSensor_TalonFX.vi"("error in (no error)"=w182, "pidLoopIdx"=w200, "Talon FX Feedback Device"=w201, "PhoenixMotorControlDevRef"=w183) -> ("error out"=w172:errorcluster, "PhoenixMotorControlDevRef"=w174:T20)  [unwired: 6 in]
            n57 = call <vilib>:"CTRE_Phoenix_MotorControl_SetSelectedSensorPosition.vi"("error in (no error)"=w172, "New Sensor Position"=0, "PhoenixMotorControlDevRef"=w174) -> ("error out"=w171:errorcluster, "PhoenixMotorControlDevRef"=w173:T20)  [unwired: 7 in]
            n58 = call <vilib>:"CTRE_Phoenix_MotorControl_ConfigClosedLoopConstants.vi"("PhoenixMotorControlDevRef"=w173, "slotIdx"=w192, "P"=w187, "I"=w186, "D"=w185, "error in (no error)"=w171, "F"=w193) -> ("PhoenixMotorControlDevRef"=w180:T20, "error out"=w179:errorcluster)  [unwired: 7 in]
            n59 = call <vilib>:"CTRE_Phoenix_MotorControl_SetSensorPhase.vi"("error in (no error)"=w179, "PhaseSensor"=FALSE, "PhoenixMotorControlDevRef"=w180) -> ("error out"=w196:errorcluster, "PhoenixMotorControlDevRef"=w197:T20)  [unwired: 7 in]
            n60 = call <vilib>:"CTRE_Phoenix_MotorControl_SetNeutralMode.vi"("error in (no error)"=w196, "Motor Control Neutral Mode"=CTRE_Phoenix_MotorControl_NeutralMode."Override to Brake", "PhoenixMotorControlDevRef"=w197) -> ("error out"=w176:errorcluster, "PhoenixMotorControlDevRef"=w177:T20)  [unwired: 7 in]
            n61 = call <vilib>:"CTRE_Phoenix_MotorControl_ConfigStatorCurrentLimit.vi"("error in (no error)"=w176, "Stator Current Limit Configuration"=T8 {"Enable?"=TRUE, "Current Limit"=35.0, "Threshold Current"=40.0, "Threshold Time"=1.0}, "PhoenixMotorControlDevRef"=w177) -> ("error out"=w190:errorcluster, "PhoenixMotorControlDevRef"=w189:T20)  [unwired: 7 in]
            n62 = call <vilib>:"CTRE_Phoenix_MotorControl_RefNumRegistrySet.vi"("error in (no error)"=w190, "refnum name"=w199, "PhoenixMotorControlDevRef"=w189) -> ("error out"=w170:errorcluster)  [unwired: 7 in, 1 out]
          }
        }
        frame "Talon FX, P6" {
          n63 = for {
            tunnel: w207 -> [w227] mode=indexing
            tunnel: [w215] -> w204 mode=indexing
            tunnel: [w211] -> w206
            w220 = u16 0 items=["RotorSensor", "RemoteCANcoder", "RemotePigeon2_Yaw", "RemotePigeon2_Pitch", "RemotePigeon2_Roll", "FusedCANcoder", "SyncCANcoder"] ("FeedbackFeedbackSensorSource")
            w221 = u16 1 items=["Coast", "Brake"] ("MotorOutputNeutralMode")
            w217 = 0.0  # D
            w218 = 0.0  # I
            w219 = 0.03  # P
            n64 = Unbundle(w227) -> (w226:i32, "Invert Type"=w216:T3, w223:string)
            n65 = call <vilib>:"TalonFX_open.vi"("CANbus Name"="8020Canivore" ("CAN Bus"), "Device ID"=w226) -> ("error out"=w214:errorcluster, "DeviceReference 2"=w222:T25)  [unwired: 8 in]
            n66 = Bundle By Name(cluster=T6 {"Future Proof Configs"=FALSE, "MotorOutputInverted"=0, "MotorOutputNeutralMode"=0, "MotorOutputDutyCycleNeutralDeadband"=0.0, "MotorOutputPeakForwardDutyCycle"=1.0, "MotorOutputPeakReverseDutyCycle"=-1.0, "MotorOutputControlTimesyncFreqHz"=0.0, "CurrentLimitsStatorCurrentLimit"=120.0, "CurrentLimitsStatorCurrentLimitEnable"=TRUE, "CurrentLimitsSupplyCurrentLimit"=70.0, "CurrentLimitsSupplyCurrentLimitEnable"=TRUE, "CurrentLimitsSupplyCurrentLowerLimit"=40.0, "CurrentLimitsSupplyCurrentLowerTime"=1.0, "VoltageSupplyVoltageTimeConstant"=0.0, "VoltagePeakForwardVoltage"=16.0, "VoltagePeakReverseVoltage"=-16.0, "TorqueCurrentPeakForwardTorqueCurrent"=800.0, "TorqueCurrentPeakReverseTorqueCurrent"=-800.0, "TorqueCurrentTorqueNeutralDeadband"=0.0, "FeedbackFeedbackRotorOffset"=0.0, "FeedbackSensorToMechanismRatio"=1.0, "FeedbackRotorToSensorRatio"=1.0, "FeedbackFeedbackSensorSource"=0, "FeedbackFeedbackRemoteSensorID"=0, "FeedbackVelocityFilterTimeConstant"=0.0, "DifferentialSensorsDifferentialSensorSource"=0, "DifferentialSensorsDifferentialTalonFXSensorID"=0, "DifferentialSensorsDifferentialRemoteSensorID"=0, "DifferentialConstantsPeakDifferentialDutyCycle"=2.0, "DifferentialConstantsPeakDifferentialVoltage"=32.0, "DifferentialConstantsPeakDifferentialTorqueCurrent"=1600.0, "OpenLoopRampsDutyCycleOpenLoopRampPeriod"=0.0, "OpenLoopRampsVoltageOpenLoopRampPeriod"=0.0, "OpenLoopRampsTorqueOpenLoopRampPeriod"=0.0, "ClosedLoopRampsDutyCycleClosedLoopRampPeriod"=0.0, "ClosedLoopRampsVoltageClosedLoopRampPeriod"=0.0, "ClosedLoopRampsTorqueClosedLoopRampPeriod"=0.0, "HardwareLimitSwitchForwardLimitType"=0, "HardwareLimitSwitchForwardLimitAutosetPositionEnable"=FALSE, "HardwareLimitSwitchForwardLimitAutosetPositionValue"=0.0, "HardwareLimitSwitchForwardLimitEnable"=TRUE, "HardwareLimitSwitchForwardLimitSource"=0, "HardwareLimitSwitchForwardLimitRemoteSensorID"=0, "HardwareLimitSwitchReverseLimitType"=0, "HardwareLimitSwitchReverseLimitAutosetPositionEnable"=FALSE, "HardwareLimitSwitchReverseLimitAutosetPositionValue"=0.0, "HardwareLimitSwitchReverseLimitEnable"=TRUE, "HardwareLimitSwitchReverseLimitSource"=0, "HardwareLimitSwitchReverseLimitRemoteSensorID"=0, "AudioBeepOnBoot"=TRUE, "AudioBeepOnConfig"=TRUE, "AudioAllowMusicDurDisable"=FALSE, "SoftwareLimitSwitchForwardSoftLimitEnable"=FALSE, "SoftwareLimitSwitchReverseSoftLimitEnable"=FALSE, "SoftwareLimitSwitchForwardSoftLimitThreshold"=0.0, "SoftwareLimitSwitchReverseSoftLimitThreshold"=0.0, "MotionMagicMotionMagicCruiseVelocity"=0.0, "MotionMagicMotionMagicAcceleration"=0.0, "MotionMagicMotionMagicJerk"=0.0, "MotionMagicMotionMagicExpo_kV"=0.12, "MotionMagicMotionMagicExpo_kA"=0.1, "CustomParamsCustomParam0"=0, "CustomParamsCustomParam1"=0, "ClosedLoopGeneralContinuousWrap"=FALSE, "Slot0kP"=0.0, "Slot0kI"=0.0, "Slot0kD"=0.0, "Slot0kS"=0.0, "Slot0kV"=0.0, "Slot0kA"=0.0, "Slot0kG"=0.0, "Slot0GravityType"=0, "Slot0StaticFeedforwardSign"=0, "Slot1kP"=0.0, "Slot1kI"=0.0, "Slot1kD"=0.0, "Slot1kS"=0.0, "Slot1kV"=0.0, "Slot1kA"=0.0, "Slot1kG"=0.0, "Slot1GravityType"=0, "Slot1StaticFeedforwardSign"=0, "Slot2kP"=0.0, "Slot2kI"=0.0, "Slot2kD"=0.0, "Slot2kS"=0.0, "Slot2kV"=0.0, "Slot2kA"=0.0, "Slot2kG"=0.0, "Slot2GravityType"=0, "Slot2StaticFeedforwardSign"=0} ("DeviceConfiguration"), "Slot0kP"=w219, "Slot0kI"=w218, "Slot0kD"=w217, "FeedbackFeedbackSensorSource"=w220, "MotorOutputNeutralMode"=w221, "MotorOutputInverted"=w216, "CurrentLimitsStatorCurrentLimitEnable"=TRUE, "CurrentLimitsStatorCurrentLimit"=35.0) -> (w215:T6)
            n67 = call <vilib>:"TalonFXConfigurator.vi"("error in"=w214, "DeviceConfiguration"=w215, "DeviceReference"=w222) -> ("error out"=w213:errorcluster)  [unwired: 8 in]
            n68 = call-poly <vilib>:"TalonFXSet.vi"("error in (no error)"=w213, "SetPosition"=0.0, "DeviceReference"=w222) -> ("error out"=w212:errorcluster)  [unwired: 8 in]
            n69 = call <vilib>:"Phoenix6_Device_RefNumRegistrySet.vi"("error in (no error)"=w212, "refnum name"=w223, "DeviceReference"=w222) -> ("error out"=w211:errorcluster)  [unwired: 7 in, 1 out]
          }
          n70 = To Variant(anything=w204) -> (Variant=w203:variant)
          n71 = call-poly <vilib>:"NT Write Value.vi"("variant"=w203, "name"="Drive/P6 Drv Config") -> ()  [unwired: 9 in, 1 out]
        }
        frame "SPARK MAX" {
          n72 = for {
            tunnel: w229 -> [w255] mode=indexing
            tunnel: [w254] -> w228
            n73 = Unbundle(w255) -> (w257:i32, "Invert Type"=w259:T3, w256:string)
            n74 = Number To Boolean Array(number=w259) -> (Boolean array=w260:bool[])
            n75 = Index Array(array=w260) -> (element=w258:bool)  [unwired: 1 in]
            n76 = call-poly <vilib>:"SPARK Open.vi"("Invert"=w258, "Device Number"=w257) -> ("error out"=w232:errorcluster, "MotorControlDeviceRef"=w233:T20)  [unwired: 8 in]
            n77 = call-poly <vilib>:"SPARK Configure Closed Loop.vi"("error in"=w232, "Feedback Sensor (Primary Encoder)"=SPARK_Feedback_Sensor."Primary Encoder", "MotorControlDeviceRef in"=w233) -> ("error out"=w238:errorcluster, "MotorControlDeviceRef out"=w240:T20)  [unwired: 7 in]
            n78 = call <vilib>:"SPARK Set Sensor Position.vi"("Sensor (Primary Encoder)"=enum16{"Primary Encoder", "Alt/Ext Encoder"}."Primary Encoder", "error in"=w238, "Position"=0.0, "MotorControlDeviceRef"=w240) -> ("error out"=w236:errorcluster, "MotorControlDeviceRef"=w237:T20)  [unwired: 6 in]
            n79 = call-poly <vilib>:"SPARK Configure Closed Loop.vi"("error in"=w236, "PID Gains"=T12 {"kP"=0.00015, "kI"=0.0, "kD"=0.0}, "MotorControlDeviceRef in"=w237) -> ("error out"=w250:errorcluster, "MotorControlDeviceRef out"=w251:T20)  [unwired: 7 in]
            n80 = call-poly <vilib>:"SPARK Configure Closed Loop.vi"("error in (no error)"=w250, "Compensated Nominal Voltage"=12.0, "Voltage Mode (Disabled)"=Closed_Loop_Voltage_Mode."Voltage Compensation", "MotorControlDeviceRef in"=w251) -> ("error out"=w244:errorcluster, "MotorControlDeviceRef out"=w245:T20)  [unwired: 6 in]
            n81 = call-poly <vilib>:"SPARK Configure Closed Loop.vi"("error in (no error)"=w244, "MotorControlDeviceRef in"=w245) -> ("error out"=w242:errorcluster, "MotorControlDeviceRef out"=w243:T20)  [unwired: 8 in]
            n82 = call-poly <vilib>:"SPARK Configure Basic.vi"("error in (no error)"=w242, "Idle Mode"=Spark_MAX_Idle_Mode."Brake", "MotorControlDeviceRef in"=w243) -> ("error out"=w246:errorcluster, "MotorControlDeviceRef out"=w247:T20)  [unwired: 7 in]
            n83 = call-poly <vilib>:"SPARK Configure Power.vi"("error in (no error)"=w246, "Primay Current Limit (80A)"=40.0, "MotorControlDeviceRef in"=w247) -> ("error out"=w230:errorcluster, "MotorControlDeviceRef out"=w231:T20)  [unwired: 7 in]
            n84 = call <vilib>:"WPI_MotorControlRefNum Registry Set.vi"("error in (no error)"=w230, "refnum name"=w256, "MotorControlDevRef"=w231) -> ("error out"=w254:errorcluster)  [unwired: 7 in, 1 out]
          }
        }
      }
      n85 = case shown="\"Talon FX, P6\"" w152 {
        tunnel: w166 -> [w262 w310 w331]
        tunnel: w167 -> [_ _ _]
        tunnel: w154 -> [w261 w309 w330]
        frame "Talon FX, P5", Default {
          n86 = for {
            tunnel: w262 -> [w305] mode=indexing
            tunnel: w261 -> [w269]
            w270 = 2048.0  # ticks per rev
            w281 = 1023.0  # Max Output
            w293 = 0  # slotIdx
            w282 = 0.0  # D
            w283 = 0.0  # I
            w284 = 0.06  # P
            w289 = 0  # pidLoopIdx
            w304 = T19 1 items=["Integrated Sensor"=1, "Sensor Sum (S0 + S1)"=9, "Sensor Difference (D0 - D1)"=10, "Remote Source 0"=11, "Remote Source 1"=12, "None"=14, "Software Emulated"=15] ("Talon FX Feedback Device")
            n87 = Unbundle(w305) -> (w302:i32, "Invert Type"=w279:T3, w303:string)
            n88 = call <vilib>:"CTRE_Phoenix_TalonFX_Open.vi"("Device Number"=w302, "CAN Bus"="8020Canivore") -> ("error out"=w287:errorcluster, "PhoenixMotorControlDevRef"=w288:T20)  [unwired: 8 in]
            n89 = call <vilib>:"CTRE_Phoenix_MotorControl_SetInverted_TalonFX.vi"("error in (no error)"=w287, "Invert Type"=w279, "PhoenixMotorControlDevRef"=w288) -> ("error out"=w285:errorcluster, "PhoenixMotorControlDevRef"=w286:T20)  [unwired: 7 in]
            n90 = Multiply(x=w269, y=w270) -> (x*y=w272:dbl[])
            n91 = Divide(x=w272, y=10.0) -> (x/y=w268:dbl[])
            n92 = call <vilib>:"CTRE_Phoenix_MotorControl_ConfigSelectedFeedbackSensor_TalonFX.vi"("error in (no error)"=w285, "pidLoopIdx"=w289, "Talon FX Feedback Device"=w304, "PhoenixMotorControlDevRef"=w286) -> ("error out"=w275:errorcluster, "PhoenixMotorControlDevRef"=w277:T20)  [unwired: 6 in]
            n93 = Index Array(array=w268) -> (element #1=w267:dbl, element #2=w266:dbl, element #3=w265:dbl)  [unwired: 3 in]
            n94 = Reciprocal(x=w265) -> (1/x=w273:dbl)
            n95 = To Long Integer(number=w267) -> (32bit integer=w264:i32)
            n96 = To Long Integer(number=w266) -> (32bit integer=w263:i32)
            n97 = call <vilib>:"CTRE_Phoenix_MotorControl_SetSelectedSensorPosition.vi"("error in (no error)"=w275, "New Sensor Position"=0, "PhoenixMotorControlDevRef"=w277) -> ("error out"=w274:errorcluster, "PhoenixMotorControlDevRef"=w276:T20)  [unwired: 7 in]
            n98 = Multiply(x=w273, y=w281) -> (x*y=w280:dbl)
            n99 = call <vilib>:"CTRE_Phoenix_MotorControl_ConfigClosedLoopConstants.vi"("PhoenixMotorControlDevRef"=w276, "slotIdx"=w293, "P"=w284, "I"=w283, "D"=w282, "error in (no error)"=w274, "F"=w280) -> ("PhoenixMotorControlDevRef"=w300:T20, "error out"=w301:errorcluster)  [unwired: 7 in]
            n100 = call <vilib>:"CTRE_Phoenix_MotorControl_ConfigMotionMagic.vi"("error in (no error)"=w301, "Acceleration"=w263, "Cruise Velocity"=w264, "PhoenixMotorControlDevRef"=w300) -> ("error out"=w299:errorcluster, "PhoenixMotorControlDevRef"=w298:T20)  [unwired: 6 in]
            n101 = call <vilib>:"CTRE_Phoenix_MotorControl_SetSensorPhase.vi"("error in (no error)"=w299, "PhaseSensor"=FALSE, "PhoenixMotorControlDevRef"=w298) -> ("error out"=w296:errorcluster, "PhoenixMotorControlDevRef"=w297:T20)  [unwired: 7 in]
            n102 = call <vilib>:"CTRE_Phoenix_MotorControl_SetNeutralMode.vi"("error in (no error)"=w296, "Motor Control Neutral Mode"=CTRE_Phoenix_MotorControl_NeutralMode."Override to Brake", "PhoenixMotorControlDevRef"=w297) -> ("error out"=w292:errorcluster, "PhoenixMotorControlDevRef"=w291:T20)  [unwired: 7 in]
            n103 = call <vilib>:"CTRE_Phoenix_MotorControl_RefNumRegistrySet.vi"("error in (no error)"=w292, "refnum name"=w303, "PhoenixMotorControlDevRef"=w291) -> ()  [unwired: 7 in, 2 out]
          }
        }
        frame "Talon FX, P6" {
          n104 = for {
            tunnel: w310 -> [w329] mode=indexing
            tunnel: w309 -> [w320]
            tunnel: [w311] -> w307 mode=indexing
            w321 = u16 0 items=["RotorSensor", "RemoteCANcoder", "RemotePigeon2_Yaw", "RemotePigeon2_Pitch", "RemotePigeon2_Roll", "FusedCANcoder", "SyncCANcoder"] ("FeedbackFeedbackSensorSource")
            w322 = u16 1 items=["Coast", "Brake"] ("MotorOutputNeutralMode")
            w317 = 0.0  # D
            w318 = 0.0  # I
            w319 = 0.1  # P
            n105 = Unbundle(w329) -> (w327:i32, "Invert Type"=w316:T3, w324:string)
            n106 = Index Array(array=w320) -> (element #3=w328:dbl)  [unwired: 3 in, 2 out]
            n107 = Reciprocal(x=w328) -> ()  [unwired: 1 out]
            n108 = call <vilib>:"TalonFX_open.vi"("CANbus Name"="8020Canivore" ("CAN Bus"), "Device ID"=w327) -> ("error out"=w315:errorcluster, "DeviceReference 2"=w323:T25)  [unwired: 8 in]
            n109 = Bundle By Name(cluster=T6 {"Future Proof Configs"=FALSE, "MotorOutputInverted"=0, "MotorOutputNeutralMode"=0, "MotorOutputDutyCycleNeutralDeadband"=0.0, "MotorOutputPeakForwardDutyCycle"=1.0, "MotorOutputPeakReverseDutyCycle"=-1.0, "MotorOutputControlTimesyncFreqHz"=0.0, "CurrentLimitsStatorCurrentLimit"=120.0, "CurrentLimitsStatorCurrentLimitEnable"=TRUE, "CurrentLimitsSupplyCurrentLimit"=70.0, "CurrentLimitsSupplyCurrentLimitEnable"=TRUE, "CurrentLimitsSupplyCurrentLowerLimit"=40.0, "CurrentLimitsSupplyCurrentLowerTime"=1.0, "VoltageSupplyVoltageTimeConstant"=0.0, "VoltagePeakForwardVoltage"=16.0, "VoltagePeakReverseVoltage"=-16.0, "TorqueCurrentPeakForwardTorqueCurrent"=800.0, "TorqueCurrentPeakReverseTorqueCurrent"=-800.0, "TorqueCurrentTorqueNeutralDeadband"=0.0, "FeedbackFeedbackRotorOffset"=0.0, "FeedbackSensorToMechanismRatio"=1.0, "FeedbackRotorToSensorRatio"=1.0, "FeedbackFeedbackSensorSource"=0, "FeedbackFeedbackRemoteSensorID"=0, "FeedbackVelocityFilterTimeConstant"=0.0, "DifferentialSensorsDifferentialSensorSource"=0, "DifferentialSensorsDifferentialTalonFXSensorID"=0, "DifferentialSensorsDifferentialRemoteSensorID"=0, "DifferentialConstantsPeakDifferentialDutyCycle"=2.0, "DifferentialConstantsPeakDifferentialVoltage"=32.0, "DifferentialConstantsPeakDifferentialTorqueCurrent"=1600.0, "OpenLoopRampsDutyCycleOpenLoopRampPeriod"=0.0, "OpenLoopRampsVoltageOpenLoopRampPeriod"=0.0, "OpenLoopRampsTorqueOpenLoopRampPeriod"=0.0, "ClosedLoopRampsDutyCycleClosedLoopRampPeriod"=0.0, "ClosedLoopRampsVoltageClosedLoopRampPeriod"=0.0, "ClosedLoopRampsTorqueClosedLoopRampPeriod"=0.0, "HardwareLimitSwitchForwardLimitType"=0, "HardwareLimitSwitchForwardLimitAutosetPositionEnable"=FALSE, "HardwareLimitSwitchForwardLimitAutosetPositionValue"=0.0, "HardwareLimitSwitchForwardLimitEnable"=TRUE, "HardwareLimitSwitchForwardLimitSource"=0, "HardwareLimitSwitchForwardLimitRemoteSensorID"=0, "HardwareLimitSwitchReverseLimitType"=0, "HardwareLimitSwitchReverseLimitAutosetPositionEnable"=FALSE, "HardwareLimitSwitchReverseLimitAutosetPositionValue"=0.0, "HardwareLimitSwitchReverseLimitEnable"=TRUE, "HardwareLimitSwitchReverseLimitSource"=0, "HardwareLimitSwitchReverseLimitRemoteSensorID"=0, "AudioBeepOnBoot"=TRUE, "AudioBeepOnConfig"=TRUE, "AudioAllowMusicDurDisable"=FALSE, "SoftwareLimitSwitchForwardSoftLimitEnable"=FALSE, "SoftwareLimitSwitchReverseSoftLimitEnable"=FALSE, "SoftwareLimitSwitchForwardSoftLimitThreshold"=0.0, "SoftwareLimitSwitchReverseSoftLimitThreshold"=0.0, "MotionMagicMotionMagicCruiseVelocity"=0.0, "MotionMagicMotionMagicAcceleration"=0.0, "MotionMagicMotionMagicJerk"=0.0, "MotionMagicMotionMagicExpo_kV"=0.12, "MotionMagicMotionMagicExpo_kA"=0.1, "CustomParamsCustomParam0"=0, "CustomParamsCustomParam1"=0, "ClosedLoopGeneralContinuousWrap"=FALSE, "Slot0kP"=0.0, "Slot0kI"=0.0, "Slot0kD"=0.0, "Slot0kS"=0.0, "Slot0kV"=0.0, "Slot0kA"=0.0, "Slot0kG"=0.0, "Slot0GravityType"=0, "Slot0StaticFeedforwardSign"=0, "Slot1kP"=0.0, "Slot1kI"=0.0, "Slot1kD"=0.0, "Slot1kS"=0.0, "Slot1kV"=0.0, "Slot1kA"=0.0, "Slot1kG"=0.0, "Slot1GravityType"=0, "Slot1StaticFeedforwardSign"=0, "Slot2kP"=0.0, "Slot2kI"=0.0, "Slot2kD"=0.0, "Slot2kS"=0.0, "Slot2kV"=0.0, "Slot2kA"=0.0, "Slot2kG"=0.0, "Slot2GravityType"=0, "Slot2StaticFeedforwardSign"=0} ("DeviceConfiguration"), "Slot0kP"=w319, "Slot0kI"=w318, "Slot0kD"=w317, "FeedbackFeedbackSensorSource"=w321, "MotorOutputNeutralMode"=w322, "MotorOutputInverted"=w316) -> (w311:T6)
            n110 = call <vilib>:"TalonFXConfigurator.vi"("error in"=w315, "DeviceConfiguration"=w311, "DeviceReference"=w323) -> ("error out"=w314:errorcluster)  [unwired: 8 in]
            n111 = call-poly <vilib>:"TalonFXSet.vi"("error in (no error)"=w314, "SetPosition"=0.0, "DeviceReference"=w323) -> ("error out"=w313:errorcluster)  [unwired: 8 in]
            n112 = call <vilib>:"Phoenix6_Device_RefNumRegistrySet.vi"("error in (no error)"=w313, "refnum name"=w324, "DeviceReference"=w323) -> ()  [unwired: 7 in, 2 out]
          }
          n113 = To Variant(anything=w307) -> (Variant=w306:variant)
          n114 = call-poly <vilib>:"NT Write Value.vi"("variant"=w306, "name"="Drive/P6 Str Config") -> ()  [unwired: 9 in, 1 out]
        }
        frame "SPARK MAX" {
          n115 = for {
            tunnel: w331 -> [w357] mode=indexing
            tunnel: w330 -> [w355]
            n116 = Unbundle(w357) -> (w359:i32, "Invert Type"=w361:T3, w358:string)
            n117 = Number To Boolean Array(number=w361) -> (Boolean array=w362:bool[])
            n118 = Index Array(array=w362) -> (element=w360:bool)  [unwired: 1 in]
            n119 = Index Array(array=w355) -> (element #1=w336:dbl, element #2=w337:dbl, element #3=w356:dbl)  [unwired: 3 in]
            n120 = call-poly <vilib>:"SPARK Open.vi"("Invert"=w360, "Device Number"=w359) -> ("error out"=w332:errorcluster, "MotorControlDeviceRef"=w333:T20)  [unwired: 8 in]
            n121 = Reciprocal(x=w356) -> ()  [unwired: 1 out]
            n122 = call-poly <vilib>:"SPARK Configure Closed Loop.vi"("error in"=w332, "Feedback Sensor (Primary Encoder)"=SPARK_Feedback_Sensor."Primary Encoder", "MotorControlDeviceRef in"=w333) -> ("error out"=w342:errorcluster, "MotorControlDeviceRef out"=w344:T20)  [unwired: 7 in]
            n123 = call <vilib>:"SPARK Set Sensor Position.vi"("Sensor (Primary Encoder)"=enum16{"Primary Encoder", "Alt/Ext Encoder"}."Primary Encoder", "error in"=w342, "Position"=0.0, "MotorControlDeviceRef"=w344) -> ("error out"=w340:errorcluster, "MotorControlDeviceRef"=w341:T20)  [unwired: 6 in]
            n124 = call-poly <vilib>:"SPARK Configure Closed Loop.vi"("error in"=w340, "PID Gains"=T12 {"kP"=0.07, "kI"=0.0, "kD"=0.0}, "MotorControlDeviceRef in"=w341) -> ("error out"=w351:errorcluster, "MotorControlDeviceRef out"=w352:T20)  [unwired: 7 in]
            n125 = call-poly <vilib>:"SPARK Configure Closed Loop.vi"("error in (no error)"=w351, "Compensated Nominal Voltage"=12.0, "Voltage Mode (Disabled)"=Closed_Loop_Voltage_Mode."Voltage Compensation", "MotorControlDeviceRef in"=w352) -> ("error out"=w348:errorcluster, "MotorControlDeviceRef out"=w349:T20)  [unwired: 6 in]
            n126 = call-poly <vilib>:"SPARK Configure Closed Loop.vi"("error in (no error)"=w348, "Max Acceleration"=w337, "Max Velocity"=w336, "MotorControlDeviceRef in"=w349) -> ("error out"=w346:errorcluster, "MotorControlDeviceRef out"=w347:T20)  [unwired: 6 in]
            n127 = call-poly <vilib>:"SPARK Configure Basic.vi"("error in (no error)"=w346, "Idle Mode"=Spark_MAX_Idle_Mode."Brake", "MotorControlDeviceRef in"=w347) -> ("error out"=w334:errorcluster, "MotorControlDeviceRef out"=w335:T20)  [unwired: 7 in]
            n128 = call <vilib>:"WPI_MotorControlRefNum Registry Set.vi"("error in (no error)"=w334, "refnum name"=w358, "MotorControlDevRef"=w335) -> ()  [unwired: 7 in, 2 out]
          }
        }
      }
      n129 = for {
        tunnel: w165 -> [w370] mode=indexing
        w371 = T26 267264 items=["SensorData"=267264, "VbatAndFaults"=267328] ("CANcoder Status Frame")
        n130 = Unbundle(w370) -> ("Device Number"=w369:u8, w368:string)
        n131 = call <vilib>:"CTRE_Phoenix_CANcoder_Open.vi"("Device Number"=w369, "CAN Bus"="8020Canivore") -> ("error out"=w363:errorcluster, "CTRE_CANcoder_DeviceRef"=w366:T27)  [unwired: 8 in]
        n132 = call <vilib>:"CTRE_Phoenix_CANcoder_ConfigSensorInitializationStrategy.vi"("error in"=w363, "Sensor Initialization Strategy"=CTRE_Phoenix_CANcoder_SensorInitializationStrategy."Boot To Absolute Position", "CTRE_CANcoder_DeviceRef"=w366) -> ("error out"=w364:errorcluster, "CTRE_CANcoder_DeviceRef"=w365:T27)  [unwired: 7 in]
        n133 = call <vilib>:"CTRE_Phoenix_CANcoder_SetStatusFrameRate.vi"("error in (no error)"=w364, "Period (ms)"=u8 20, "CANcoder Status Frame"=w371, "CTRE_CANcoder_DeviceRef"=w365) -> ("error out"=w374:errorcluster, "CTRE_CANcoder_DeviceRef"=w373:T27)  [unwired: 6 in]
        n134 = call <vilib>:"CTRE_Phoenix_CANcoder_RefNumRegistrySet.vi"("error in (no error)"=w374, "refnum name"=w368, "CTRE_CANcoder_DeviceRef"=w373) -> ()  [unwired: 7 in, 2 out]
      }
      n135 = call <vilib>:"CTRE_Phoenix_Pigeon2_Open.vi"("Device Number"=u8 11, "canbus"="8020Canivore") -> ("error out"=w156:errorcluster, "PigeonIMUDevRef"=w157:T28)  [unwired: 8 in]
      n136 = call <vilib>:"CTRE_PigeonIMU_SetYaw.vi"("error in (no error)"=w156, "TareType (SetValue)"=w159, "Value"=0.0, "PigeonIMUDevRef"=w157) -> ("error out"=w161:errorcluster, "PigeonIMUDevRef"=w162:T28)  [unwired: 6 in]
      n137 = call <vilib>:"CTRE_PigeonIMU_RefNumRegistrySet.vi"("error in (no error)"=w161, "refnum name"="Pigeon 2.0", "PigeonIMUDevRef"=w162) -> ()  [unwired: 7 in, 2 out]
    }
  }
  n138 = global write "SWERVE_DRIVE_GLOBALS.vi" "Drv Gear Ratio"(w28) -> ()
  n139 = global write "SWERVE_DRIVE_GLOBALS.vi" "Str Gear Ratio"(w4) -> ()
  n140 = global write "SWERVE_DRIVE_GLOBALS.vi" "Wheel Diameter IN"(w3) -> ()
  n141 = call <vilib>:"Translation2d_Create.vi"("Y"=0.2625, "X"=0.2625) -> ("TRANSLATION"=w21:T30)  [unwired: 9 in]
  n142 = call <vilib>:"Translation2d_Create.vi"("Y"=-0.2625, "X"=0.2625) -> ("TRANSLATION"=w20:T30)  [unwired: 9 in]
  n143 = call <vilib>:"Translation2d_Create.vi"("Y"=0.2625, "X"=-0.2625) -> ("TRANSLATION"=w19:T30)  [unwired: 9 in]
  n144 = call <vilib>:"Translation2d_Create.vi"("Y"=-0.2625, "X"=-0.2625) -> ("TRANSLATION"=w14:T30)  [unwired: 9 in]
  n145 = Build Array(w21, w20, w19, w14) -> (w18:T30[])
  n146 = call <vilib>:"SwerveKinematics_NewX.vi"("Wheels"=w18) -> ("SWERVE_DRIVE_KINEMATICS"=w57:T31)  [unwired: 10 in]
  n147 = call "SWERVE_DRIVE_KINEMATIC_FGV.vi"("in SWERVE_DRIVE_KINEMATICS"=w57, "WRITE"=TRUE) -> ()  [unwired: 9 in, 1 out]
  n148 = call <vilib>:"Rotation2d_CreateAngleDegrees.vi"("Angle_Degrees"=w45) -> ("ROTATION"=w46:T33)  [unwired: 10 in]
  n149 = call <vilib>:"Rotation2d_CreateAngleDegrees.vi"("Angle_Degrees"=w41) -> ("ROTATION"=w42:T33)  [unwired: 10 in]
  n150 = call <vilib>:"Rotation2d_CreateAngleDegrees.vi"("Angle_Degrees"=w38) -> ("ROTATION"=w39:T33)  [unwired: 10 in]
  n151 = call <vilib>:"Rotation2d_CreateAngleDegrees.vi"("Angle_Degrees"=w35) -> ("ROTATION"=w36:T33)  [unwired: 10 in]
  n152 = call <vilib>:"SwerveModulePosition_New.vi"("ROTATION"=w46, "Distance"=w47) -> ("SWERVE_DRIVE_MODULE_POSITION"=w44:T34)  [unwired: 9 in]
  n153 = call <vilib>:"SwerveModulePosition_New.vi"("ROTATION"=w42, "Distance"=w43) -> ("SWERVE_DRIVE_MODULE_POSITION"=w34:T34)  [unwired: 9 in]
  n154 = call <vilib>:"SwerveModulePosition_New.vi"("ROTATION"=w39, "Distance"=w40) -> ("SWERVE_DRIVE_MODULE_POSITION"=w33:T34)  [unwired: 9 in]
  n155 = call <vilib>:"SwerveModulePosition_New.vi"("ROTATION"=w36, "Distance"=w37) -> ("SWERVE_DRIVE_MODULE_POSITION"=w32:T34)  [unwired: 9 in]
  n156 = Build Array(w44, w34, w33, w32) -> (w53:T34[])
  n157 = call <vilib>:"Conv_Deg_Radians.vi"("Degress"=w51) -> ("Radians"=w52:dbl)  [unwired: 10 in]
  n158 = call <vilib>:"Rotation2d_CreateAngle.vi"("Angle"=w50) -> ("ROTATION"=w56:T33)  [unwired: 10 in]
  n159 = call <vilib>:"Pose2d_New.vi"("Heading"=w52, "Y"=w49, "X"=w48) -> ("out POSe"=w59:T35)  [unwired: 8 in]
  n160 = call "SWERVE_ODOM_ABS_INITIAL_POSE_FGV.vi"("in INITIAL_POSE2D"=w59, "WRITE"=TRUE) -> ()  [unwired: 9 in, 1 out]
  n161 = call "SWERVE_ODOM_ABS_BEGIN.vi"("VisionMeasurementStdDevs"=w55, "StateStdDevs"=w54, "in SWERVE_DRIVE_KINEMATICS"=w57, "out POSe"=w59, "ROTATION"=w56, "Swerve Module Pos"=w53) -> ()  [unwired: 6 in]
  "error out" <- "error in"
